vi "KGN Set Temp.vi"(7 "Temperature":dbl[](array[numeric]) format="%.2f", 8 "Fehler (Eingang, kein Fehler)":errorcluster, 9 "Info Cluster":T1, 10 "VISA-Referenz (Eingang)":refnum<visa-resource-name>, 11 "device (Eingang)":u32) -> (0 "Fehler (Ausgang)":errorcluster, 1 "Info Cluster out":T1, 2 "VISA-Referenz (Ausgang)":refnum<visa-resource-name>, 3 "dup device (Ausgang)":u32, 4 "Kommandos gesendet":string)   [LabVIEW 2020, in "Linearisierung v2.lvlib" / "Gasteiler.lvlib" / "HovaCAL_Interface.lvlib" / "KGN.lvlib" / "KGN GUI Set.lvlib"]
uses:
  KGN GUI Set.lvlib
  Controls/Info Cluster.ctl
  set/set.lvlib
  Controls/Controls.lvlib
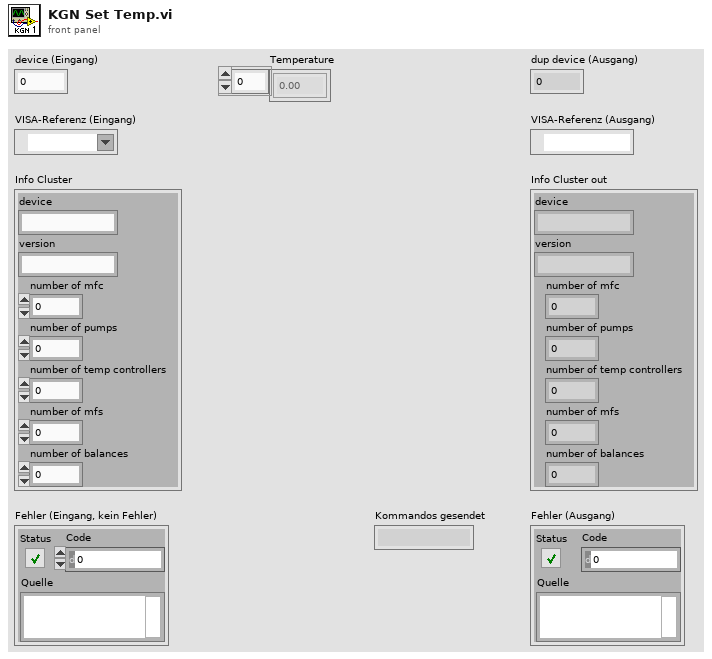
[diagram p1: front panel]
types:
  T1 = typedef "Linearisierung v2.lvlib/Gasteiler.lvlib/HovaCAL_Interface.lvlib/Controls.lvlib/Info Cluster.ctl" = cluster{"device":string, "version":string, "number of mfc":i32, "number of pumps":i32, "number of temp controllers":i32, "number of mfs":i32, "number of balances":i32}
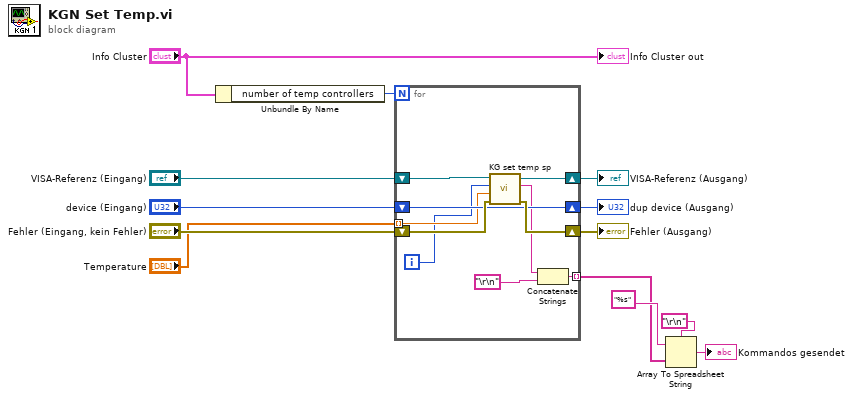
[diagram p0: block diagram]
diagram:
  n1 = Unbundle By Name("Info Cluster") -> ("number of temp controllers"=w7:i32)
  n2 = for {
    N: w7 -> [_]
    tunnel: "Temperature" -> [w20] mode=indexing
    shift-right: [w21] -> w9
    shift-left: "device (Eingang)" -> [w21]
    shift-right: [w22] -> w10
    shift-left: "Fehler (Eingang, kein Fehler)" -> [w23]
    shift-right: [w17] -> w5
    shift-left: "VISA-Referenz (Eingang)" -> [w18]
    tunnel: [w14] -> w2 mode=indexing
    i -> [w19]
    n3 = call "KG set temp sp.vi"("Fehler (Eingang, kein Fehler)"=w23, "temp"=w20, "controller"=w19, "VISA-Ressourcenname"=w18) -> ("Fehler (Ausgang)"=w22:errorcluster, "Kommando gesendet"=w15:string, "VISA-Ressourcenname (Ausgang)"=w17:refnum<visa-resource-name>)  [unwired: 5 in]
    n4 = Concatenate Strings(w15, "\r\n") -> (w14:string)
  }
  "dup device (Ausgang)" <- w9
  "Fehler (Ausgang)" <- w10
  "VISA-Referenz (Ausgang)" <- w5
  n5 = Array To Spreadsheet String(delimiter (Tab)="\r\n", array=w2, 3:"%s" ("Format-String")) -> (spreadsheet string=→"Kommandos gesendet":string)
  "Info Cluster out" <- "Info Cluster"
